vi "Finish.vi"   [LabVIEW 2012]
doc: "This VI is called just before exiting. It is expected to close I/O refnum, save collected data, etc."
uses:
  <vilib>/Rock Robotics/WPI/Compressor/WPI_CompressorGetSetRefNum.vi
  <vilib>/Rock Robotics/WPI/Joystick/WPI_JoystickGetSetRefNum.vi
  <vilib>/Rock Robotics/WPI/RobotDrive/WPI_RobotDriveGetSetRefNum.vi
types:
  T1 = typedef "WPI_SolenoidDevRef.ctl" = cluster{"DevStatus":errorcluster, "Solenoid Module":T2, "Forward Solenoid Channel":T3, "Reverse Solenoid Channel":T3}
  T2 = typedef "FPGA_TypedefSolenoidModule.ctl" = enum16{"Solenoid Module 1", "Solenoid Module 2"}
  T3 = typedef "WPI_SolenoidChannel.ctl" = enum8{"Solenoid 1", "Solenoid 2", "Solenoid 3", "Solenoid 4", "Solenoid 5", "Solenoid 6", "Solenoid 7", "Solenoid 8", "Invalid"}
  T4 = typedef "WPI_MotorControlDeviceRef.ctl" = cluster{"DeviceStatus":errorcluster, "Type":enum16{"PWM", "CAN"}, "PWM":cluster{"Digital Module":T5, "PWM Channel":T6, "DeadBand":T7}, "CAN":cluster{"Device Number":u8, "Control Mode":T8, "Semaphore":T9, "Max Vout":dbl}, "Invert":bool, "TransformRef":T10, "InvTransformRef":T10}
  T5 = typedef "FPGA_TypedefDigitalModule.ctl" = enum16{"Digital Module 1", "Digital Module 2"}
  T6 = typedef "FPGA_DIOPWMChannel.ctl" = enum8{"PWM 1", "PWM 2", "PWM 3", "PWM 4", "PWM 5", "PWM 6", "PWM 7", "PWM 8", "PWM 9", "PWM 10", "Invalid"}
  T7 = typedef "WPI_PWMDeadband.ctl" = cluster{"Name":string, "maxPositivePwm":i32, "minPositivePwm":i32, "centerPwm":i32, "maxNegativePwm":i32, "minNegativePwm":i32, "angularRange":u16}
  T8 = typedef "WPI_CANJaguar_ControlMode.ctl" = enum8{"Percent VBus", "Current", "Speed", "Position", "Voltage"}
  T9 = typedef "Semaphore RefNum" = refnum<k1>
  T10 = typedef "WPI_PWMTransform_ConPane.ctl" = refnum<vi>
  T11 = typedef "WPI_EncoderDevRef.ctl" = cluster{"DevStatus":errorcluster, "EncoderIndex":T12, "CounterIndex":T13, "DistancePerCount":dbl, "Decoding Type":T14}
  T12 = typedef "FPGA_EncoderIdx.ctl" = enum8{"Enc 0", "Enc 1", "Enc 2", "Enc 3", "Invalid"}
  T13 = typedef "FPGA_CounterCtrSystemIndex.ctl" = enum8{"Ctr 0", "Ctr 1", "Ctr 2", "Ctr 3", "Ctr 4", "Ctr 5", "Ctr 6", "Ctr 7", "Invalid"}
  T14 = typedef "WPI_EncoderType.ctl" = enum16{"1x", "2x", "4x"}
  T15 = typedef "WPI_RelayDevRef.ctl" = cluster{"DevStatus":errorcluster, "Relay Channel":T16, "Digital Module":T5, "Relay Direction":T17}
  T16 = typedef "FPGA_DIORelayChannel.ctl" = enum8{"Relay 1", "Relay 2", "Relay 3", "Relay 4", "Relay 5", "Relay 6", "Relay 7", "Relay 8", "Invalid"}
  T17 = typedef "WPI_RelayDirection.ctl" = enum16{"Both directions", "Forward only", "Reverse only"}
  T18 = typedef "WPI_CompressorDevRef.ctl" = cluster{"DevStatus":errorcluster, "DigitalInputDevRef":T19, "RelayDevRef":T15}
  T19 = typedef "WPI_DigitalInputDevRef.ctl" = cluster{"DevStatus":errorcluster, "DIO Channel":T20, "Digital Module":T5}
  T20 = typedef "FPGA_DIOChannel.ctl" = enum8{"DIO 1", "DIO 2", "DIO 3", "DIO 4", "DIO 5", "DIO 6", "DIO 7", "DIO 8", "DIO 9", "DIO 10", "DIO 11", "DIO 12", "DIO 13", "DIO 14", "Invalid"}
  T21 = typedef "WPI_UltrasonicDeviceRef.ctl" = cluster{"DevStatus":errorcluster, "Ping Digital Module":T5, "Echo Digital Module":T5, "Ping Channel":T20, "Echo Channel":T20, "CntIndex":T13}
  T22 = typedef "WPI_JoystickDevRef.ctl" = cluster{"Device":T23}
  T23 = typedef "WPI_JoystickDeviceEnum.ctl" = enum16{"USB 1", "USB 2", "USB 3", "USB 4", "Kinect 1", "Kinect 2"}
  T24 = typedef "WPI_RobotDriveDevRef.ctl" = cluster{"DevStatus":errorcluster, "Motors[]":T4[], "Square Inputs":bool, "Max Output":dbl, "Isochronous":bool}
  T25 = typedef "WPI_CameraDevRef.ctl" = cluster{"Camera Address":string, "CameraStatus":errorcluster, "Acquire Image Notifier":refnum<notifier>}
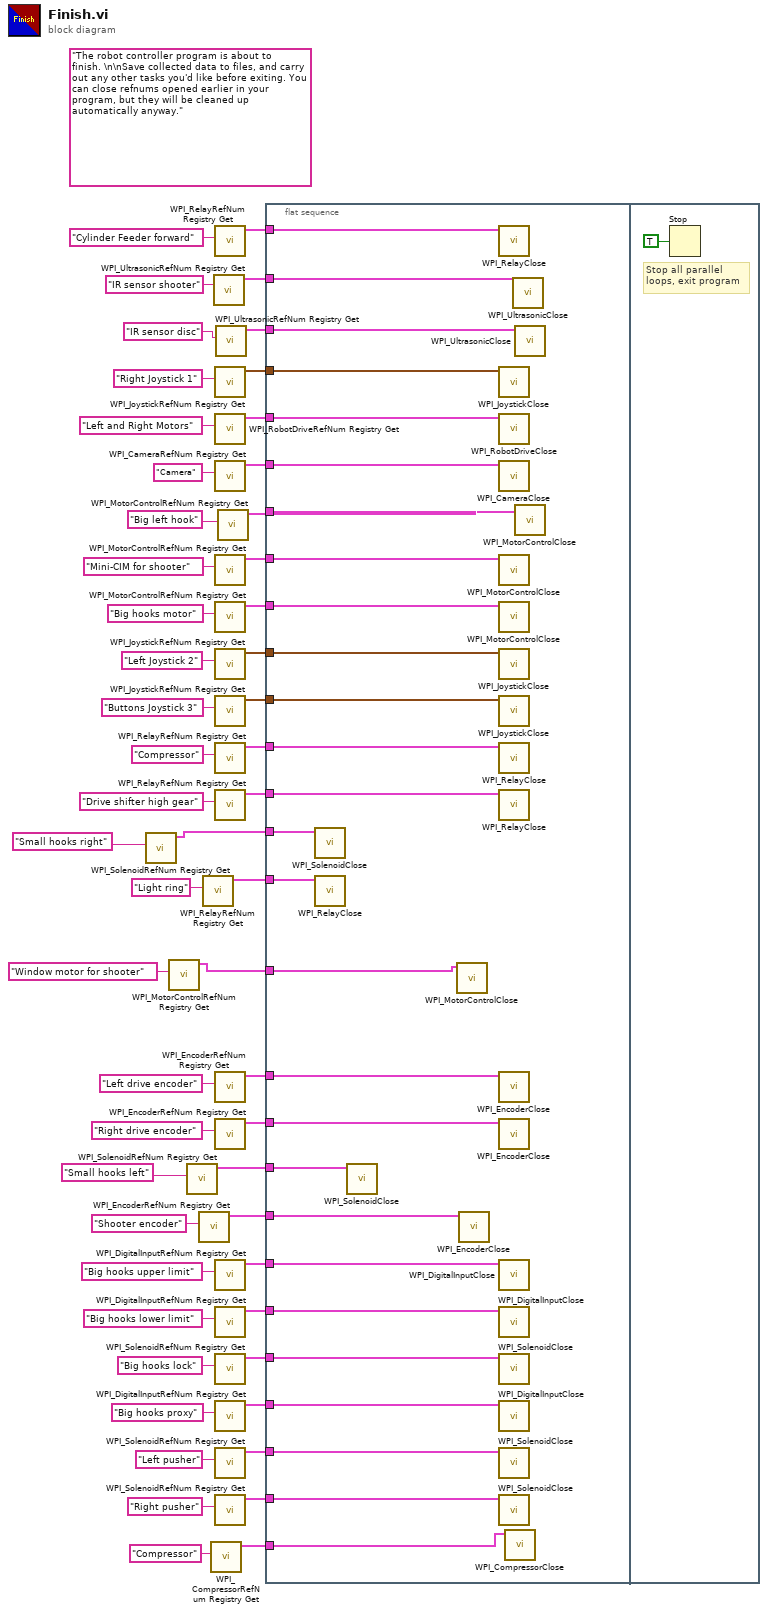
[diagram p0: block diagram]
diagram:
  (unwired) "The robot controller program is about to finish. \n\nSave collected data to files, and carry out any other tasks you'd like before exiting. You can close refnums opened earlier in your program, but they will be cleaned up automatically anyway."
  n1 = call <vilib>:"WPI_SolenoidRefNum Registry Get.vi"("refnum name"="Small hooks right") -> ("SolenoidDevRef"=w1:T1)  [unwired: 9 in, 1 out]
  n2 = call <vilib>:"WPI_MotorControlRefNum Registry Get.vi"("refnum name"="Window motor for shooter") -> ("MotorControlDevRef"=w9:T4)  [unwired: 9 in, 1 out]
  n3 = call <vilib>:"WPI_SolenoidRefNum Registry Get.vi"("refnum name"="Small hooks left") -> ("SolenoidDevRef"=w3:T1)  [unwired: 9 in, 1 out]
  n4 = call <vilib>:"WPI_EncoderRefNum Registry Get.vi"("refnum name"="Shooter encoder") -> ("EncoderDevRef"=w7:T11)  [unwired: 9 in, 1 out]
  n5 = call <vilib>:"WPI_RelayRefNum Registry Get.vi"("refnum name"="Light ring") -> ("RelayDevRef"=w5:T15)  [unwired: 9 in, 1 out]
  n6 = call <vilib>:"WPI_CompressorRefNum Registry Get.vi"("refnum name"="Compressor") -> ("CompressorDevRef"=w16:T18)  [unwired: 9 in, 1 out]
  n7 = call <vilib>:"WPI_UltrasonicRefNum Registry Get.vi"("refnum name"="IR sensor shooter") -> ("UltrasonicDevRef"=w11:T21)  [unwired: 9 in, 1 out]
  n8 = call <vilib>:"WPI_RelayRefNum Registry Get.vi"("refnum name"="Cylinder Feeder forward") -> ("RelayDevRef"=w35:T15)  [unwired: 9 in, 1 out]
  n9 = call <vilib>:"WPI_JoystickRefNum Registry Get.vi"("refnum name"="Right Joystick 1") -> ("JoystickDevRef"=w51:T22)  [unwired: 1 in, 9 out]
  n10 = call <vilib>:"WPI_RobotDriveRefNum Registry Get.vi"("refnum name"="Left and Right Motors") -> ("RobotDriveDevRef"=w52:T24)  [unwired: 1 in, 9 out]
  n11 = call <vilib>:"WPI_CameraRefNum Registry Get.vi"("refnum name"="Camera") -> ("CameraDevRef"=w50:T25)  [unwired: 1 in, 9 out]
  n12 = call <vilib>:"WPI_MotorControlRefNum Registry Get.vi"("refnum name"="Mini-CIM for shooter") -> ("MotorControlDevRef"=w44:T4)  [unwired: 9 in, 1 out]
  n13 = call <vilib>:"WPI_MotorControlRefNum Registry Get.vi"("refnum name"="Big hooks motor") -> ("MotorControlDevRef"=w43:T4)  [unwired: 9 in, 1 out]
  n14 = call <vilib>:"WPI_JoystickRefNum Registry Get.vi"("refnum name"="Left Joystick 2") -> ("JoystickDevRef"=w41:T22)  [unwired: 1 in, 9 out]
  n15 = call <vilib>:"WPI_JoystickRefNum Registry Get.vi"("refnum name"="Buttons Joystick 3") -> ("JoystickDevRef"=w39:T22)  [unwired: 1 in, 9 out]
  n16 = call <vilib>:"WPI_RelayRefNum Registry Get.vi"("refnum name"="Compressor") -> ("RelayDevRef"=w36:T15)  [unwired: 9 in, 1 out]
  n17 = call <vilib>:"WPI_RelayRefNum Registry Get.vi"("refnum name"="Drive shifter high gear") -> ("RelayDevRef"=w34:T15)  [unwired: 9 in, 1 out]
  n18 = call <vilib>:"WPI_EncoderRefNum Registry Get.vi"("refnum name"="Left drive encoder") -> ("EncoderDevRef"=w32:T11)  [unwired: 9 in, 1 out]
  n19 = call <vilib>:"WPI_EncoderRefNum Registry Get.vi"("refnum name"="Right drive encoder") -> ("EncoderDevRef"=w29:T11)  [unwired: 9 in, 1 out]
  n20 = call <vilib>:"WPI_DigitalInputRefNum Registry Get.vi"("refnum name"="Big hooks upper limit") -> ("DigitalInputDevRef"=w27:T19)  [unwired: 9 in, 1 out]
  n21 = call <vilib>:"WPI_DigitalInputRefNum Registry Get.vi"("refnum name"="Big hooks lower limit") -> ("DigitalInputDevRef"=w25:T19)  [unwired: 9 in, 1 out]
  n22 = call <vilib>:"WPI_SolenoidRefNum Registry Get.vi"("refnum name"="Big hooks lock") -> ("SolenoidDevRef"=w23:T1)  [unwired: 9 in, 1 out]
  n23 = call <vilib>:"WPI_DigitalInputRefNum Registry Get.vi"("refnum name"="Big hooks proxy") -> ("DigitalInputDevRef"=w21:T19)  [unwired: 9 in, 1 out]
  n24 = call <vilib>:"WPI_SolenoidRefNum Registry Get.vi"("refnum name"="Left pusher") -> ("SolenoidDevRef"=w19:T1)  [unwired: 9 in, 1 out]
  n25 = call <vilib>:"WPI_SolenoidRefNum Registry Get.vi"("refnum name"="Right pusher") -> ("SolenoidDevRef"=w17:T1)  [unwired: 9 in, 1 out]
  n26 = call <vilib>:"WPI_UltrasonicRefNum Registry Get.vi"("refnum name"="IR sensor disc") -> ("UltrasonicDevRef"=w13:T21)  [unwired: 9 in, 1 out]
  n27 = call <vilib>:"WPI_MotorControlRefNum Registry Get.vi"("refnum name"="Big left hook") -> ("MotorControlDevRef"=w47:T4)  [unwired: 9 in, 1 out]
  n28 = flat-sequence {
    tunnel: w52 -> [w81]
    tunnel: w51 -> [w80]
    tunnel: w50 -> [w79]
    tunnel: w47 -> [w78]
    tunnel: w44 -> [w77]
    tunnel: w43 -> [w76]
    tunnel: w41 -> [w75]
    tunnel: w39 -> [w74]
    tunnel: w36 -> [w73]
    tunnel: w35 -> [w72]
    tunnel: w34 -> [w71]
    tunnel: w32 -> [w70]
    tunnel: w29 -> [w69]
    tunnel: w27 -> [w68]
    tunnel: w25 -> [w67]
    tunnel: w23 -> [w66]
    tunnel: w21 -> [w65]
    tunnel: w19 -> [w64]
    tunnel: w17 -> [w63]
    tunnel: w16 -> [w62]
    tunnel: w13 -> [w61]
    tunnel: w11 -> [w60]
    tunnel: w9 -> [w59]
    tunnel: w7 -> [w58]
    tunnel: w5 -> [w57]
    tunnel: w3 -> [w56]
    tunnel: w1 -> [w55]
    frame #0 {
      n29 = call <vilib>:"WPI_SolenoidClose.vi"("SolenoidDevRef"=w55) -> ()  [unwired: 10 in, 1 out]
      n30 = call <vilib>:"WPI_RelayClose.vi"("RelayDevRef"=w57) -> ()  [unwired: 10 in, 1 out]
      n31 = call <vilib>:"WPI_SolenoidClose.vi"("SolenoidDevRef"=w56) -> ()  [unwired: 10 in, 1 out]
      n32 = call <vilib>:"WPI_MotorControlClose.vi"("MotorControlDevRef"=w59) -> ()  [unwired: 10 in, 1 out]
      n33 = call <vilib>:"WPI_EncoderClose.vi"("EncoderDevRef"=w58) -> ()  [unwired: 10 in, 1 out]
      n34 = call <vilib>:"WPI_RelayClose.vi"("RelayDevRef"=w72) -> ()  [unwired: 10 in, 1 out]
      n35 = call <vilib>:"WPI_JoystickClose.vi"("JoystickDevRef"=w80) -> ()  [unwired: 11 out]
      n36 = call <vilib>:"WPI_RobotDriveClose.vi"("RobotDriveDevRef"=w81) -> ()  [unwired: 1 in, 10 out]
      n37 = call <vilib>:"WPI_CameraClose.vi"("CameraDevRef"=w79) -> ()  [unwired: 1 in, 10 out]
      n38 = call <vilib>:"WPI_MotorControlClose.vi"("MotorControlDevRef"=w77) -> ()  [unwired: 10 in, 1 out]
      n39 = call <vilib>:"WPI_MotorControlClose.vi"("MotorControlDevRef"=w76) -> ()  [unwired: 10 in, 1 out]
      n40 = call <vilib>:"WPI_JoystickClose.vi"("JoystickDevRef"=w75) -> ()  [unwired: 11 out]
      n41 = call <vilib>:"WPI_JoystickClose.vi"("JoystickDevRef"=w74) -> ()  [unwired: 11 out]
      n42 = call <vilib>:"WPI_RelayClose.vi"("RelayDevRef"=w73) -> ()  [unwired: 10 in, 1 out]
      n43 = call <vilib>:"WPI_RelayClose.vi"("RelayDevRef"=w71) -> ()  [unwired: 10 in, 1 out]
      n44 = call <vilib>:"WPI_EncoderClose.vi"("EncoderDevRef"=w70) -> ()  [unwired: 10 in, 1 out]
      n45 = call <vilib>:"WPI_EncoderClose.vi"("EncoderDevRef"=w69) -> ()  [unwired: 10 in, 1 out]
      n46 = call <vilib>:"WPI_DigitalInputClose.vi"("DigitalInputDevRef"=w68) -> ()  [unwired: 10 in, 1 out]
      n47 = call <vilib>:"WPI_DigitalInputClose.vi"("DigitalInputDevRef"=w67) -> ()  [unwired: 10 in, 1 out]
      n48 = call <vilib>:"WPI_SolenoidClose.vi"("SolenoidDevRef"=w66) -> ()  [unwired: 10 in, 1 out]
      n49 = call <vilib>:"WPI_DigitalInputClose.vi"("DigitalInputDevRef"=w65) -> ()  [unwired: 10 in, 1 out]
      n50 = call <vilib>:"WPI_SolenoidClose.vi"("SolenoidDevRef"=w64) -> ()  [unwired: 10 in, 1 out]
      n51 = call <vilib>:"WPI_SolenoidClose.vi"("SolenoidDevRef"=w63) -> ()  [unwired: 10 in, 1 out]
      n52 = call <vilib>:"WPI_CompressorClose.vi"("CompressorDevRef"=w62) -> ()  [unwired: 10 in, 1 out]
      n53 = call <vilib>:"WPI_UltrasonicClose.vi"("UltrasonicDevRef"=w60) -> ()  [unwired: 10 in, 1 out]
      n54 = call <vilib>:"WPI_UltrasonicClose.vi"("UltrasonicDevRef"=w61) -> ()  [unwired: 10 in, 1 out]
      n55 = call <vilib>:"WPI_MotorControlClose.vi"("MotorControlDevRef"=w78) -> ()  [unwired: 10 in, 1 out]
    }
    frame #1 {
      # "Stop all parallel\nloops, exit program"
      n56 = Stop(stop? (T)=TRUE ("Quit")) -> ()
    }
  }
